vi "open Port.vi"(11 "port_num":i32) -> (3 "function return":u8)   [LabVIEW 2016, in "dxl_x86_c.lvlib"]
doc: "WINDECLSPEC uint8_t openPort (int port_num);"
uses:
  dxl_x86_c.lvlib
  dxl_x86_c.dll
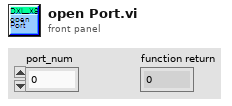
[diagram p1: front panel]
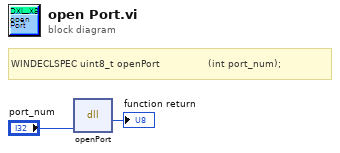
[diagram p0: block diagram]
diagram:
  # "WINDECLSPEC uint8_t openPort                (int port_num);"
  n1 = dll-call lib="C:/Users/Platform/Desktop/GITHUB/DynamixelSDK/labview/dxl_x86_c.lvlib/dxl_x86_c.*" fn="openPort"("port_num"="port_num") -> (→"function return":u8)  [unwired: 4 in, 2 out]
